vi "NTV_Compass.vi"(7 "Read(f) Write(t)":bool, 11 "Compass":T1 scale format="%.3f") -> (3 "Compass Out":T1 scale format="%.3f")   [LabVIEW 2020]
uses:
  TypeDefs/Dial_Compase heading unit circle CCW positive.ctl
  <vilib>/Rock Robotics/Network Tables/NT Read Number.vi
  <vilib>/Rock Robotics/Network Tables/NT Write Number.vi
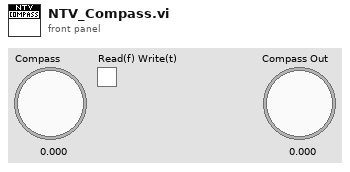
[diagram p1: front panel]
types:
  T1 = typedef "Dial_Compase heading unit circle CCW positive.ctl" = dbl
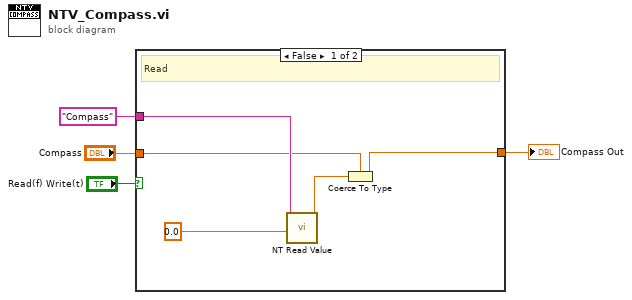
[diagram p0: block diagram]
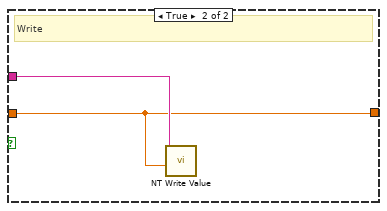
[diagram p2: hidden frame]
diagram:
  n1 = case shown="False" "Read(f) Write(t)" {
    tunnel: "Compass" -> [w7 w10]
    tunnel: "Compass" ("Name") -> [w9 w11]
    tunnel: [w8 w10] -> w1
    frame False {
      # "Read"
      n2 = call-poly <vilib>:"NT Read Value.vi"("default value"=0.0 ("Default Value"), "name"=w9) -> ("value"=w6:dbl)  [unwired: 7 in, 2 out]
      n3 = Coerce To Type(0:w6, 1:w7) -> (2:w8:T1)
    }
    frame True {
      # "Write"
      n4 = call-poly <vilib>:"NT Write Value.vi"("value"=w10, "name"=w11) -> ()  [unwired: 9 in, 1 out]
    }
  }
  "Compass Out" <- w1
